vi "FGV MODEL.vi"(7 "STATES":T1, 11 "MODEL IN":string) -> (3 "MODEL OUT":string)   [LabVIEW 2025]
uses:
  Controls/MODEL CONTROL.ctl
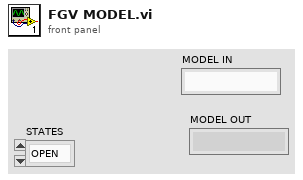
[diagram p1: front panel]
types:
  T1 = typedef "MODEL CONTROL.ctl" = enum16{"OPEN", "READ", "WRITE", "CLOSE"}
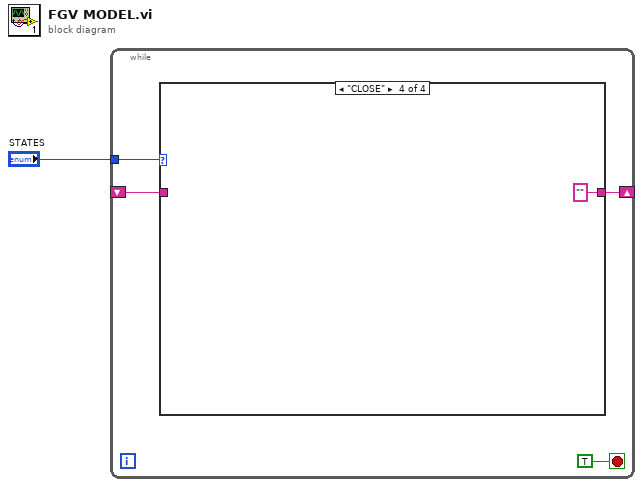
[diagram p0: block diagram]
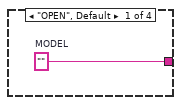
[diagram p2: hidden frame]
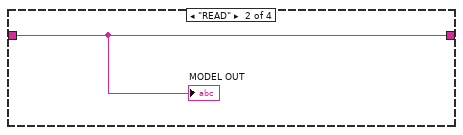
[diagram p3: hidden frame]
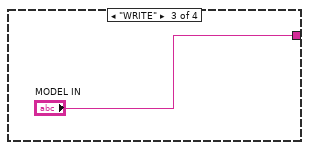
[diagram p4: hidden frame]
diagram:
  n1 = while {
    tunnel: "STATES" -> [w4]
    shift-right: [w3] -> _
    shift-left: _ -> [w2]
    stop <- TRUE stop-if-true
    n2 = case shown="\"CLOSE\"" w4 {
      tunnel: [w6 w7 "MODEL IN" "" ("MODEL IN")] -> w3
      tunnel: w2 -> [_ w7 _ _]
      frame "OPEN", Default {
        w6 = ""  # MODEL
      }
      frame "READ" {
        "MODEL OUT" <- w7
      }
      frame "WRITE" {
      }
      frame "CLOSE" {
      }
    }
  }
